vi "TesteJSON.vi"() -> ()   [LabVIEW 2019]
panel:
  out "Right Wheel Velocity":dbl
  out "Left Wheel Velocity":dbl
  in  "Parar 2":bool
  out "sorted array":cluster{"time":dbl}[](array[cluster])
  out "size(s)":i32
  out "Times 2":cluster{"time":dbl}
  out "Times":cluster{"time":dbl}
  out "Curvature":dbl
  out "Radians":dbl
  out "y":dbl
  out "x":dbl
  out "Acceleration":dbl
  out "Velocity":dbl
  out "Time":dbl
  out "x 3":dbl
  out "x 2":dbl
  out "x":dbl
  out "Acceleration":dbl
  out "Velocity":dbl
  out "Time":dbl
  out "text":string
  # "Pose"
  # "Translation"
  # "Rotation"
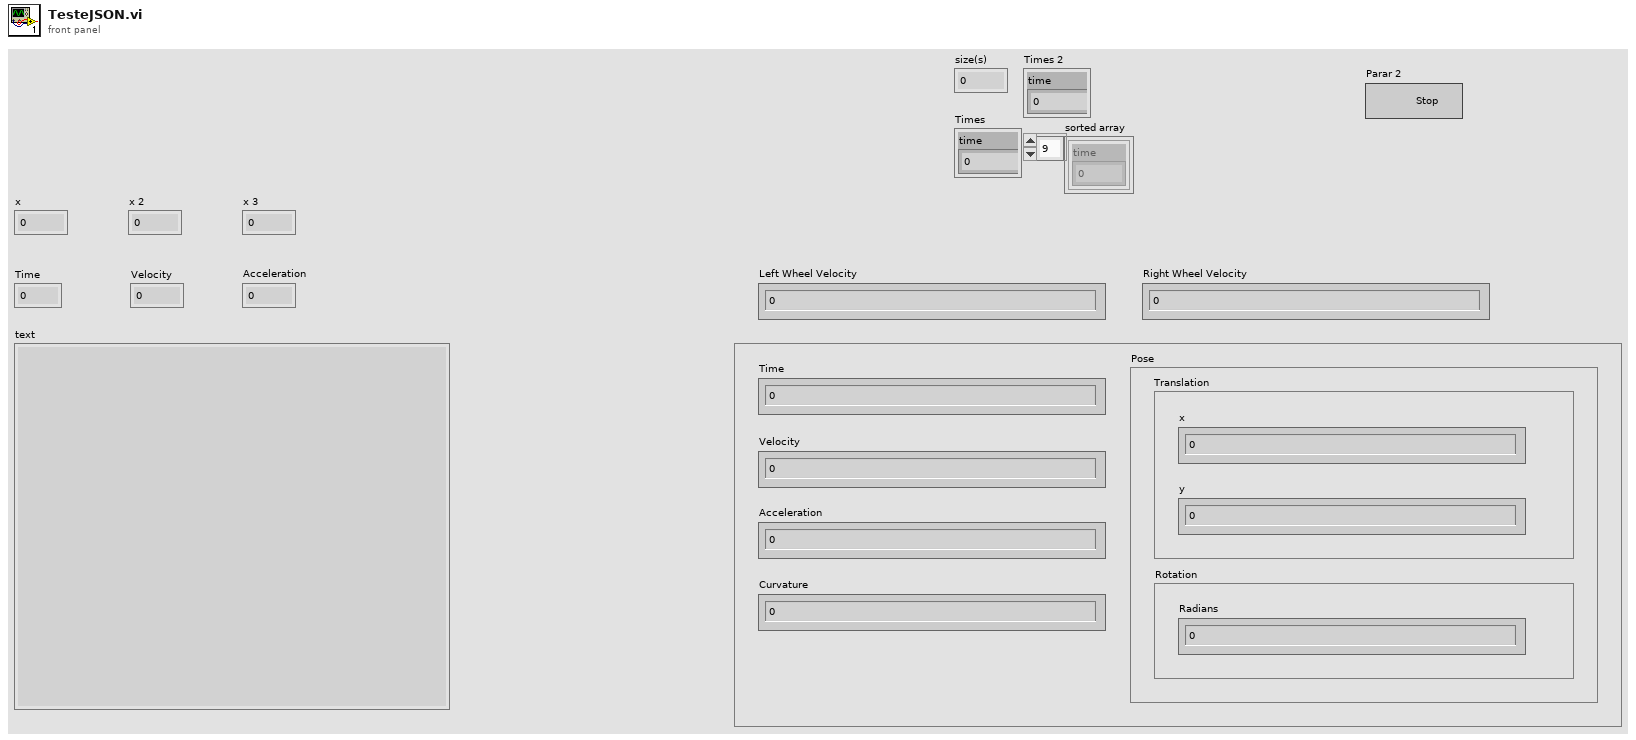
[diagram p1: front panel]
types:
  T1 = cluster{"translation":cluster{"x":dbl, "y":dbl}, "rotation":cluster{"radians":dbl}}
  T2 = cluster{"time":dbl, "acceleration":dbl, "velocity":dbl}[]
  T3 = cluster{"[0]":cluster{"time":dbl, "acceleration":dbl, "velocity":dbl}, "[1]":cluster{"time":dbl, "acceleration":dbl, "velocity":dbl}, "[2]":cluster{"time":dbl, "acceleration":dbl, "velocity":dbl}, "[3]":cluster{"time":dbl, "acceleration":dbl, "velocity":dbl}, "[4]":cluster{"time":dbl, "acceleration":dbl, "velocity":dbl}, "[5]":cluster{"time":dbl, "acceleration":dbl, "velocity":dbl}, "[6]":cluster{"time":dbl, "acceleration":dbl, "velocity":dbl}, "[7]":cluster{"time":dbl, "acceleration":dbl, "velocity":dbl}, "[8]":cluster{"time":dbl, "acceleration":dbl, "velocity":dbl}}
  T4 = cluster{"pose":cluster{"translation":cluster{"y":dbl, "x":dbl}}}[]
  T5 = cluster{"[0]":cluster{"pose":cluster{"translation":cluster{"y":dbl, "x":dbl}}}, "[1]":cluster{"pose":cluster{"translation":cluster{"y":dbl, "x":dbl}}}, "[2]":cluster{"pose":cluster{"translation":cluster{"y":dbl, "x":dbl}}}, "[3]":cluster{"pose":cluster{"translation":cluster{"y":dbl, "x":dbl}}}, "[4]":cluster{"pose":cluster{"translation":cluster{"y":dbl, "x":dbl}}}, "[5]":cluster{"pose":cluster{"translation":cluster{"y":dbl, "x":dbl}}}, "[6]":cluster{"pose":cluster{"translation":cluster{"y":dbl, "x":dbl}}}, "[7]":cluster{"pose":cluster{"translation":cluster{"y":dbl, "x":dbl}}}, "[8]":cluster{"pose":cluster{"translation":cluster{"y":dbl, "x":dbl}}}}
  T6 = cluster{"pose":cluster{"rotation":cluster{"radians":dbl}}}[]
  T7 = cluster{"curvature":dbl, "acceleration":dbl, "velocity":dbl}[]
  T8 = cluster{"curvature":dbl, "acceleration":dbl, "velocity":dbl}
  T9 = cluster{"pose":cluster{"translation":cluster{"y":dbl, "x":dbl}}}
  T10 = cluster{"pose":cluster{"rotation":cluster{"radians":dbl}}}
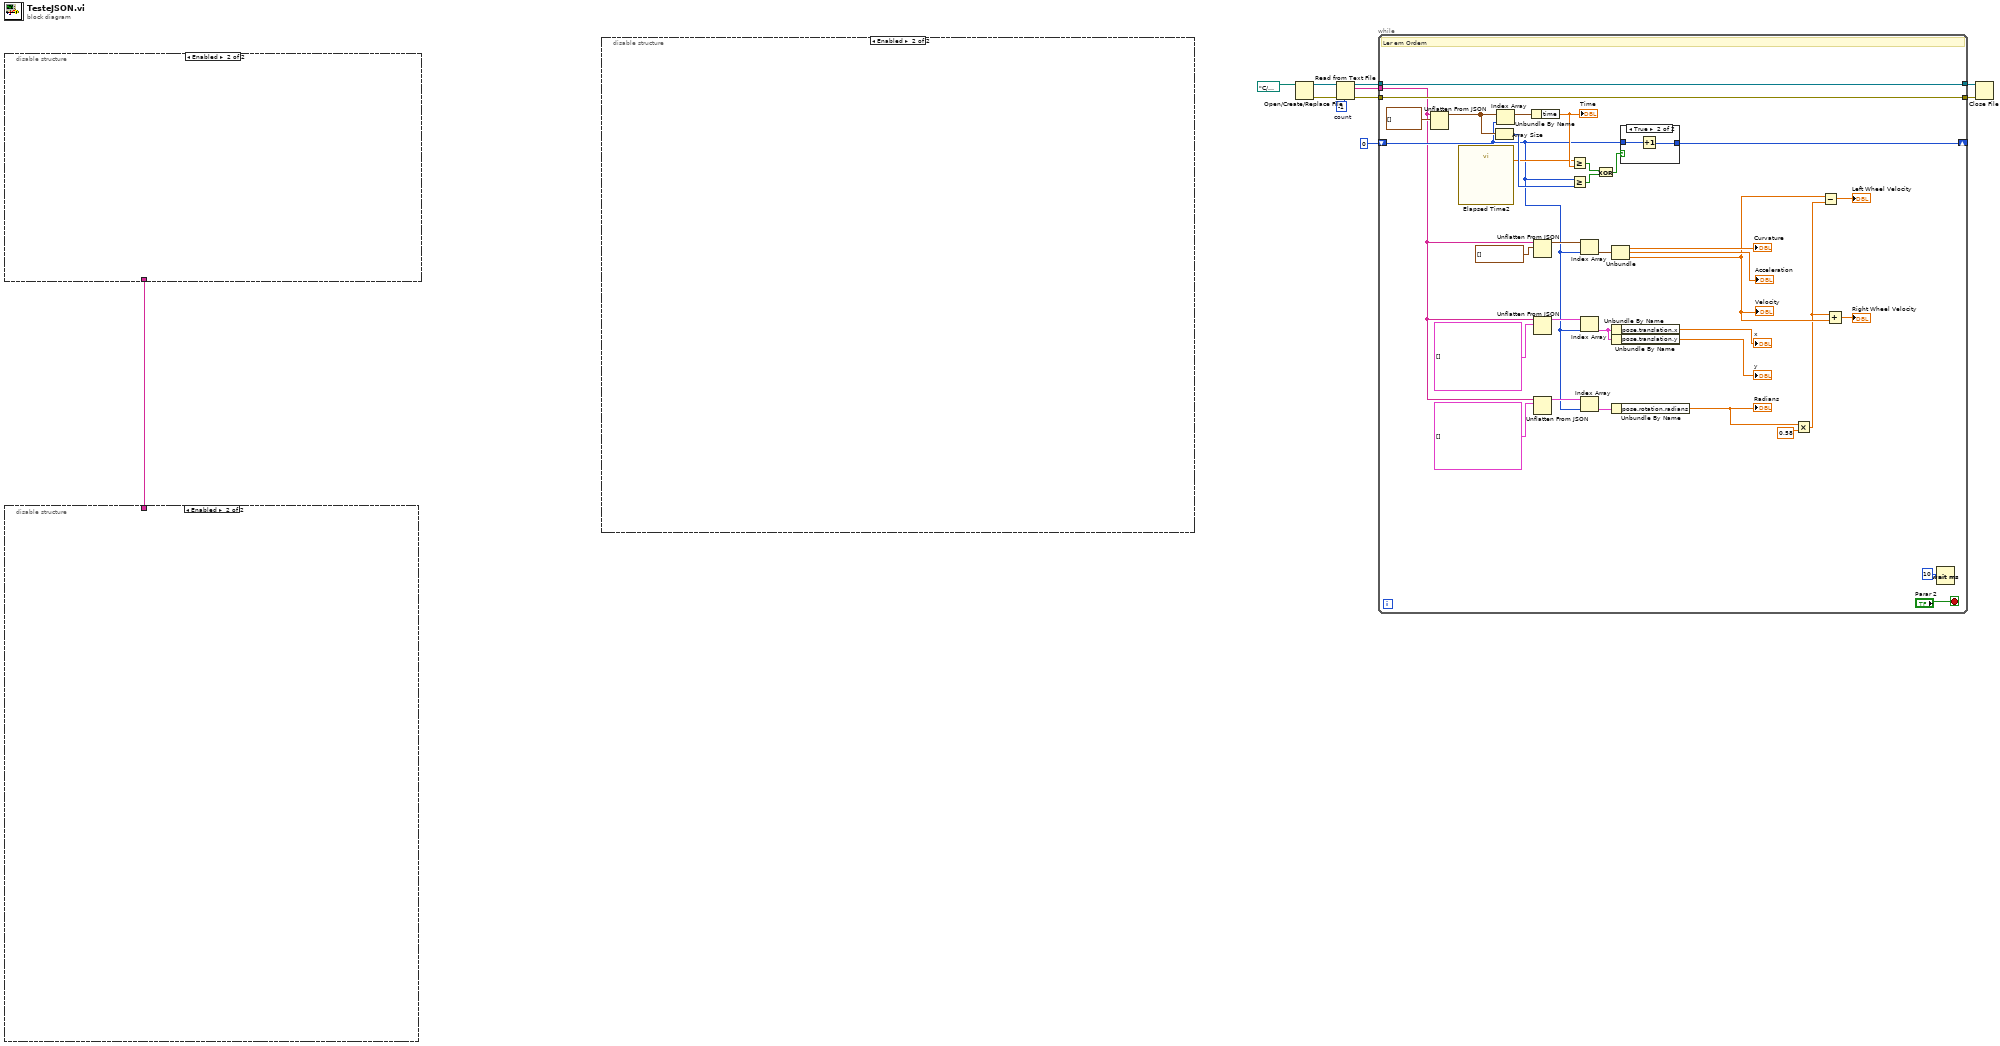
[diagram p0: block diagram]
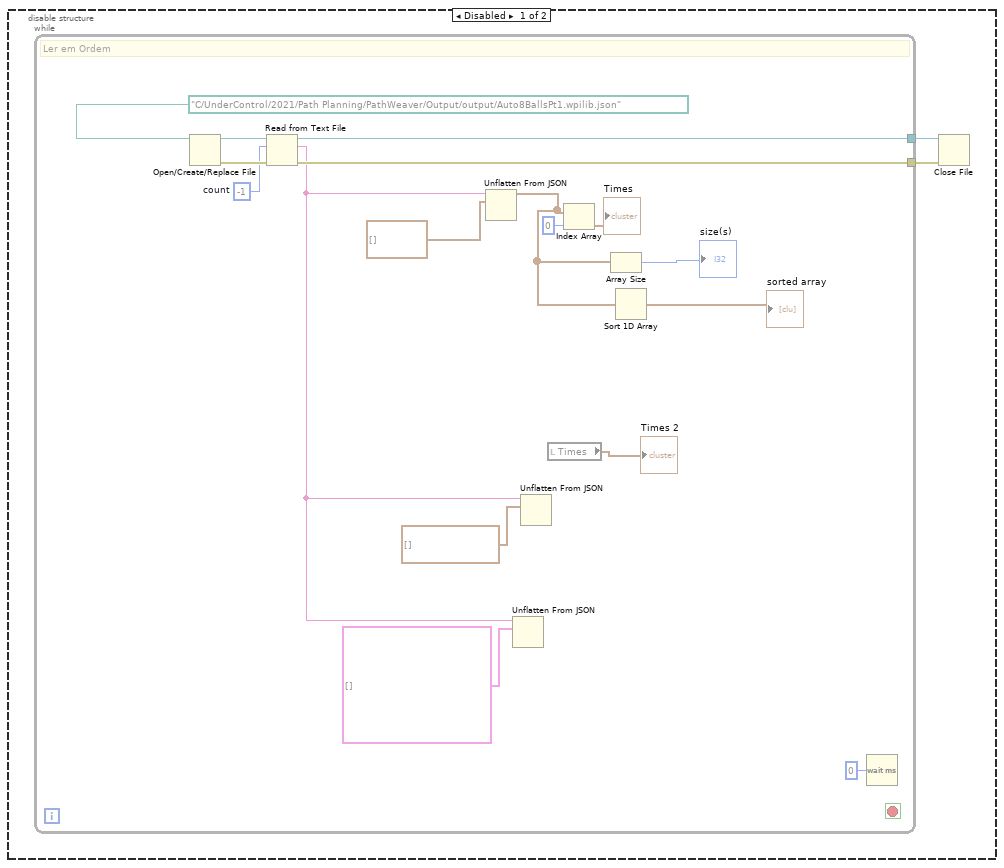
[diagram p2: hidden frame]
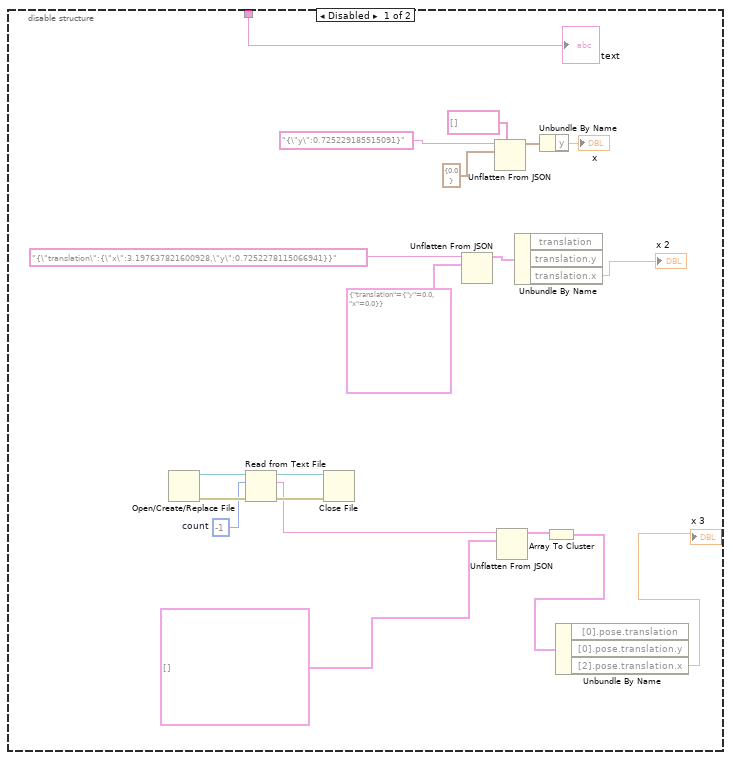
[diagram p4: hidden frame]
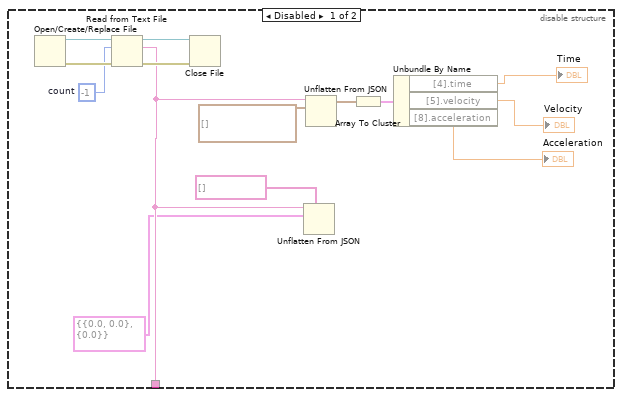
[diagram p5: hidden frame]
diagram:
  w9 = -1  # count
  n1 = disable-structure shown="Enabled" {
    disable-tunnel: [w14 _] -> w11
    frame Disabled {
      w23 = -1  # count
      n2 = Open/Create/Replace File() -> (refnum out=w24:refnum<file>, error out=w25:errorcluster)  [unwired: 6 in, 1 out]
      n3 = Read from Text File(file (use dialog)=w24, count=w23, error in=w25) -> (refnum out=w21:refnum<file>, text=w14:string, error out=w22:errorcluster)  [unwired: 1 in, 1 out]
      n4 = Close File(refnum=w21, error in=w22) -> ()  [unwired: 2 out]
      n5 = Unflatten From JSON(path=string[] [], JSON string=w14, type and defaults=T1 {"translation"={"x"=0.0, "y"=0.0}, "rotation"={"radians"=0.0}}) -> ()  [unwired: 4 in, 2 out]
      n6 = Unflatten From JSON(JSON string=w14, type and defaults=T2 []) -> (value=w16:T2)  [unwired: 5 in, 1 out]
      n7 = Array To Cluster(array=w16) -> (cluster=w19:T3)
      n8 = Unbundle By Name(w19) -> ("[4].time"=→"Time":dbl, "[5].velocity"=→"Velocity":dbl, "[8].acceleration"=→"Acceleration":dbl)
    }
    frame Enabled {
    }
  }
  n9 = disable-structure shown="Enabled" {
    disable-tunnel: w11 -> [w45 _]
    frame Disabled {
      w33 = -1  # count
      n10 = Open/Create/Replace File() -> (refnum out=w34:refnum<file>, error out=w35:errorcluster)  [unwired: 6 in, 1 out]
      n11 = Read from Text File(file (use dialog)=w34, count=w33, error in=w35) -> (refnum out=w31:refnum<file>, text=w30:string, error out=w32:errorcluster)  [unwired: 1 in, 1 out]
      n12 = Close File(refnum=w31, error in=w32) -> ()  [unwired: 2 out]
      n13 = Unflatten From JSON(JSON string="{\"translation\":{\"x\":3.197637821600928,\"y\":0.7252278115066941}}", type and defaults=cluster{"translation":cluster{"y":dbl, "x":dbl}} {"translation"={"y"=0.0, "x"=0.0}}) -> (value=w38:cluster{"translation":cluster{"y":dbl, "x":dbl}})  [unwired: 5 in, 1 out]
      n14 = Unflatten From JSON(path=string[] [], JSON string="{\"y\":0.725229185515091}", type and defaults=cluster{"y":dbl} {"y"=0.0}) -> (value=w41:cluster{"y":dbl})  [unwired: 4 in, 1 out]
      n15 = Unflatten From JSON(JSON string=w30, type and defaults=T4 []) -> (value=w28:T4)  [unwired: 5 in, 1 out]
      n16 = Unbundle By Name(w38) -> ("translation.x"=→"x 2":dbl)  [unwired: 2 out]
      n17 = Unbundle By Name(w41) -> ("y"=→"x":dbl)
      n18 = Array To Cluster(array=w28) -> (cluster=w27:T5)
      n19 = Unbundle By Name(w27) -> ("[2].pose.translation.x"=→"x 3":dbl)  [unwired: 2 out]
      "text" <- w45
    }
    frame Enabled {
    }
  }
  n20 = disable-structure shown="Enabled" {
    frame Disabled {
      n21 = while {
        tunnel: [w61] -> w47
        tunnel: [w60] -> w46
        stop <- w58 stop-if-true
        w63 = -1  # count
        # "Ler em Ordem"
        n22 = Open/Create/Replace File(file path (use dialog)=path "C:/UnderControl/2021/Path Planning/PathWeaver/Output/output/Auto8BallsPt1.wpilib.json") -> (refnum out=w64:refnum<file>, error out=w65:errorcluster)  [unwired: 5 in, 1 out]
        n23 = Read from Text File(file (use dialog)=w64, count=w63, error in=w65) -> (refnum out=w60:refnum<file>, text=w53:string, error out=w61:errorcluster)  [unwired: 1 in, 1 out]
        n24 = Unflatten From JSON(JSON string=w53, type and defaults=cluster{"time":dbl}[] []) -> (value=w49:cluster{"time":dbl}[])  [unwired: 5 in, 1 out]
        n25 = Unflatten From JSON(JSON string=w53, type and defaults=T4 []) -> ()  [unwired: 5 in, 2 out]
        n26 = Unflatten From JSON(JSON string=w53, type and defaults=T2 []) -> ()  [unwired: 5 in, 2 out]
        n27 = local read "Times"() -> (→"Times 2":cluster{"time":dbl})
        n28 = Index Array(array=w49, index=0) -> (element=→"Times":cluster{"time":dbl})
        n29 = Array Size(array=w49) -> (size(s)=→"size(s)":i32)
        n30 = Sort 1D Array(array=w49) -> (sorted array=→"sorted array":cluster{"time":dbl}[])
        n31 = Wait (ms)(milliseconds to wait=u32 0) -> ()  [unwired: 1 out]
      }
      n32 = Close File(refnum=w46, error in=w47) -> ()  [unwired: 2 out]
    }
    frame Enabled {
    }
  }
  n33 = Open/Create/Replace File(file path (use dialog)=path "C:/UnderControl/2021/Path Planning/PathWeaver/Output/output/Auto8BallsPt1.wpilib.json") -> (refnum out=w8:refnum<file>, error out=w7:errorcluster)  [unwired: 5 in, 1 out]
  n34 = Read from Text File(file (use dialog)=w8, count=w9, error in=w7) -> (refnum out=w5:refnum<file>, text=w6:string, error out=w2:errorcluster)  [unwired: 1 in, 1 out]
  n35 = while {
    tunnel: w6 -> [w76]
    tunnel: w5 -> [w96]
    tunnel: [w96] -> w4
    tunnel: [w95] -> w3
    tunnel: w2 -> [w95]
    shift-right: [w94] -> _
    shift-left: 0 ("index") -> [w77]
    stop <- "Parar 2" stop-if-true
    # "Ler em Ordem"
    n36 = Unflatten From JSON(JSON string=w76, type and defaults=cluster{"time":dbl}[] []) -> (value=w92:cluster{"time":dbl}[])  [unwired: 5 in, 1 out]
    n37 = call "Elapsed Time2"() -> ("Elapsed Time (s)"=w87:dbl)  [unwired: 12 in, 7 out]
    n38 = Array Size(array=w92) -> (size(s)=w88:i32)
    n39 = Index Array(array=w92, index=w77) -> (element=w97:cluster{"time":dbl})
    n40 = Unbundle By Name(w97) -> ("time"=w93:dbl)
    "Time" <- w93
    n41 = Unflatten From JSON(JSON string=w76, type and defaults=T7 []) -> (value=w85:T7)  [unwired: 5 in, 1 out]
    n42 = Unflatten From JSON(JSON string=w76, type and defaults=T4 []) -> (value=w82:T4)  [unwired: 5 in, 1 out]
    n43 = Unflatten From JSON(JSON string=w76, type and defaults=T6 []) -> (value=w79:T6)  [unwired: 5 in, 1 out]
    n44 = Greater Or Equal?(x=w87, y=w93) -> (x >= y?=w90:bool)
    n45 = Greater Or Equal?(x=w77, y=w88) -> (x >= y?=w91:bool)
    n46 = Index Array(array=w85, index=w77) -> (element=w84:T8)
    n47 = Index Array(array=w82, index=w77) -> (element=w81:T9)
    n48 = Index Array(array=w79, index=w77) -> (element=w78:T10)
    n49 = Exclusive Or(1:w91, 2:w90) -> (0:w89:bool)
    n50 = Unbundle(w84) -> ("curvature"=→"Curvature":dbl, "acceleration"=→"Acceleration":dbl, "velocity"=w67:dbl)
    "Velocity" <- w67
    n51 = Unbundle By Name(w81) -> ("pose.translation.x"=→"x":dbl)
    n52 = Unbundle By Name(w81) -> ("pose.translation.y"=→"y":dbl)
    n53 = Unbundle By Name(w78) -> ("pose.rotation.radians"=w70:dbl)
    "Radians" <- w70
    n54 = case shown="True" w89 {
      tunnel: [w101 w103] -> w94
      tunnel: w77 -> [w101 w102]
      frame False {
      }
      frame True {
        n55 = Increment(x=w102) -> (x+1=w103:i32)
      }
    }
    n56 = Multiply(x=w70, y=0.58) -> (x*y=w66:dbl)
    n57 = Subtract(x=w67, y=w66) -> (x-y=→"Left Wheel Velocity":dbl)
    n58 = Add(x=w66, y=w67) -> (x+y=→"Right Wheel Velocity":dbl)
    n59 = Wait (ms)(milliseconds to wait=u32 10) -> ()  [unwired: 1 out]
  }
  n60 = Close File(refnum=w4, error in=w3) -> ()  [unwired: 2 out]
